vi "Execute.vi"(8 "error in":errorcluster, 11 "Scheduler in":refnum<class "Scheduler.lvclass">) -> (0 "error out":errorcluster, 1 "Next Step?":bool, 2 "MSG":string, 3 "Scheduler out":refnum<class "Scheduler.lvclass">)   [LabVIEW 2012, in "Scheduler.lvclass"]
doc: "Execute the SEQ execute function only if we are on the day of week specified by the DOW pointer."
uses:
  Scheduler.lvclass
  Scheduler.lvclass/Scheduler.ctl
  MSR/Sequence Composition/SEQ/SEQ.lvclass
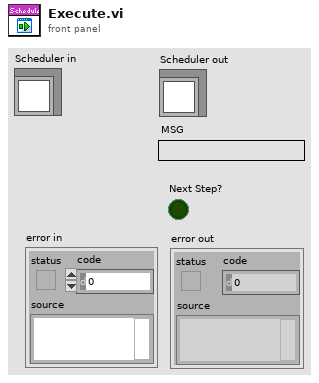
[diagram p1: front panel]
types:
  T1 = typedef "LVDateTimeRec.ctl" = cluster{"fractional second":dbl, "second":i32, "minute":i32, "hour":i32, "day of month":i32, "month":i32, "year":i32, "day of week":i32, "day of year":i32, "DST":i32}
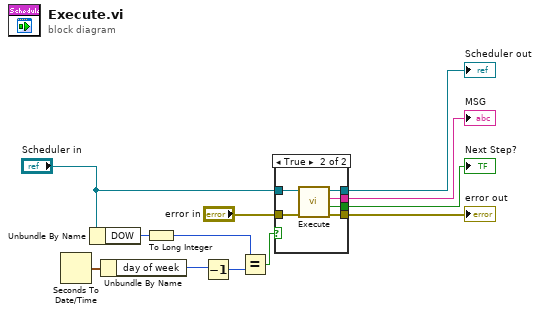
[diagram p0: block diagram]
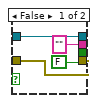
[diagram p2: hidden frame]
diagram:
  n1 = Seconds To Date/Time() -> (date time rec=w7:T1)  [unwired: 2 in]
  n2 = Unbundle By Name("Scheduler in") -> ("DOW"=w5:u8)
  n3 = Unbundle By Name(w7) -> ("day of week"=w2:i32)
  n4 = To Long Integer(number=w5) -> (32bit integer=w4:i32)
  n5 = Decrement(x=w2) -> (x-1=w1:i32)
  n6 = Equal?(x=w4, y=w1) -> (x = y?=w3:bool)
  n7 = case shown="True" w3 {
    tunnel: [w13 w22] -> w12
    tunnel: [FALSE ("Next Step?") w21] -> w11
    tunnel: ["" ("MSG") w20] -> w10
    tunnel: [w16 w19] -> w9
    tunnel: "error in" -> [w13 w18]
    tunnel: "Scheduler in" -> [w16 w17]
    frame False {
    }
    frame True {
      n8 = call-parent "Execute.vi"("error in"=w18, "SEQ in"=w17) -> ("error out"=w22:errorcluster, "Next Step?"=w21:bool, "MSG"=w20:string, "SEQ out"=w19:refnum<class "Scheduler.lvclass">)  [unwired: 6 in]
    }
  }
  "error out" <- w12
  "Scheduler out" <- w9
  "Next Step?" <- w11
  "MSG" <- w10
